vi "createILCModeFrame.vi"(8 "error in (no error)":errorcluster, 9 "TriggerIRQ":bool, 10 "WaitForTrigger":bool, 11 "ILC in":refnum<class "ILC.lvclass">) -> (0 "error out":errorcluster, 2 "Frame":T1 {"Data" format="%02x"}, 3 "ILC out":refnum<class "ILC.lvclass">)   [LabVIEW 2016, in "RTILC.lvlib" / "ILC.lvclass"]
uses:
  ILC.lvclass
  Common_RT_Modbus/DataTypes/Frame.ctl
  Common_RT_Modbus/DynamicFrameBuilder/DynamicFrameBuilder.lvclass
  ILC.lvclass/ILC.ctl
  Common_RT_Modbus/RTModbus.lvlib
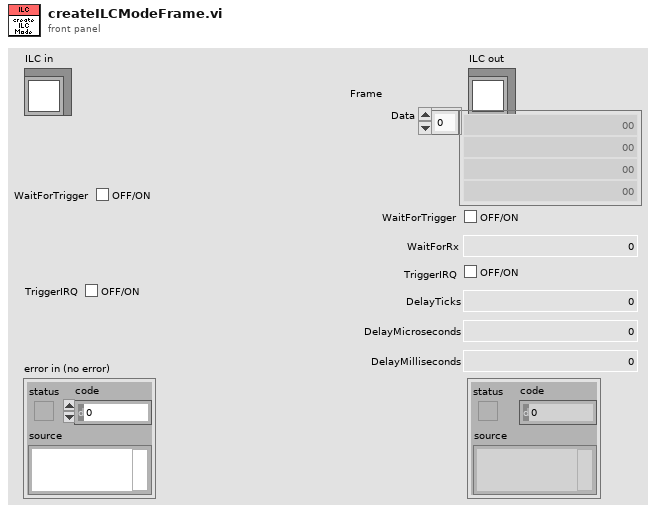
[diagram p1: front panel]
types:
  T1 = typedef "RTModbus.lvlib/Frame.ctl" = cluster{"Data":u8[], "WaitForTrigger":bool, "WaitForRx":u16, "TriggerIRQ":bool, "DelayTicks":u16, "DelayMicroseconds":u16, "DelayMilliseconds":u16}
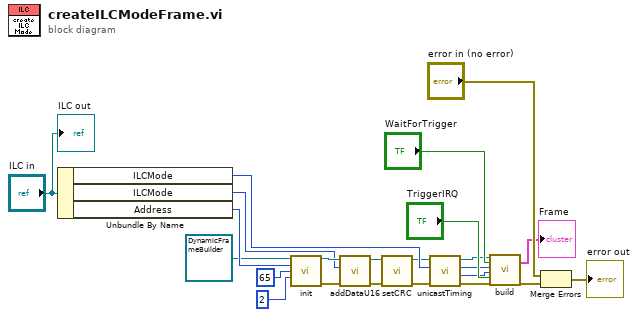
[diagram p0: block diagram]
diagram:
  n1 = Unbundle By Name("ILC in") -> ("ILCMode"=w7:u32, "ILCMode"=w16:u16, "Address"=w19:u8)
  n2 = call "init.vi"("DynamicFrameBuilder in"=refnum<class "DynamicFrameBuilder.lvclass"> refnum ("RTModbus.lvlib:DynamicFrameBuilder.lvclass"), "Address"=w19, "Function"=u8 65, "DataSize"=2) -> ("DynamicFrameBuilder out"=w17:refnum<class "DynamicFrameBuilder.lvclass">, "error out"=w15:errorcluster)  [unwired: 10 in]
  n3 = call "addDataU16.vi"("error in (no error)"=w15, "Data"=w16, "DynamicFrameBuilder in"=w17) -> ("error out"=w13:errorcluster, "DynamicFrameBuilder out"=w14:refnum<class "DynamicFrameBuilder.lvclass">)  [unwired: 7 in]
  n4 = call "setCRC.vi"("error in (no error)"=w13, "DynamicFrameBuilder in"=w14) -> ("error out"=w1:errorcluster, "DynamicFrameBuilder out"=w2:refnum<class "DynamicFrameBuilder.lvclass">)  [unwired: 8 in]
  n5 = call "unicastTiming.vi"("error in (no error)"=w1, "Latency in"=w7, "DynamicFrameBuilder in"=w2) -> ("error out"=w4:errorcluster, "WaitForRxTimeout"=w5:u16, "Latency out"=w6:u32, "DynamicFrameBuilder out"=w3:refnum<class "DynamicFrameBuilder.lvclass">)  [unwired: 5 in]
  n6 = call "build.vi"("DynamicFrameBuilder in"=w3, "WaitForTrigger"="WaitForTrigger", "Latency"=w6, "WaitForRxTimeout"=w5, "TriggerIRQ"="TriggerIRQ", "error in (no error)"=w4) -> ("Frame"=→"Frame":T1, "error out"=w9:errorcluster)  [unwired: 11 in, 1 out]
  n7 = Merge Errors("error in (no error)", w9) -> (→"error out":errorcluster)
  "ILC out" <- "ILC in"
